vi "Scale_Graph_Y2 (SubVI).vi"(10 "M [Nm]":dbl[](array[numeric]), 11 "XYGraph (Eingang)":refnum<vi>) -> ()   [LabVIEW 2014]
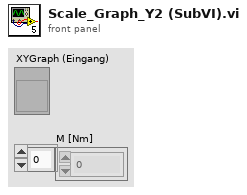
[diagram p1: front panel]
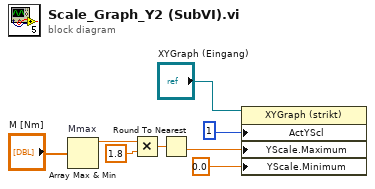
[diagram p0: block diagram]
diagram:
  n1 = Array Max & Min "Mmax"(array="M [Nm]") -> (max value=w4:dbl)  [unwired: 3 out]
  n2 = Multiply(x=w4, y=1.8) -> (x*y=w5:dbl)
  n3 = Round To Nearest(number=w5) -> (nearest integer value=w7:dbl)
  n4 = property on="Eigenschaftsknoten" class="XYGraph (strikt)"(reference="XYGraph (Eingang)", "ActYScl"=1, "YScale.Maximum"=w7, "YScale.Minimum"=0.0) -> ()  [unwired: 1 in, 2 out]
